vi "GetGlobalDefaultConfiguration.vi"(2 "DO NOT override instruments":bool, 3 "Read defaults?":bool) -> (1 "Configuration File IV":path)   [LabVIEW 2018]
uses:
  QC_MeasurementSetup.vi
  InstrControl/InstrControl.lvclass
panel:
  out "Configuration File Striptest":path
  out "Configuration File Cis":path
  out "Configuration File Stability":path
  out "Configuration File CV":path
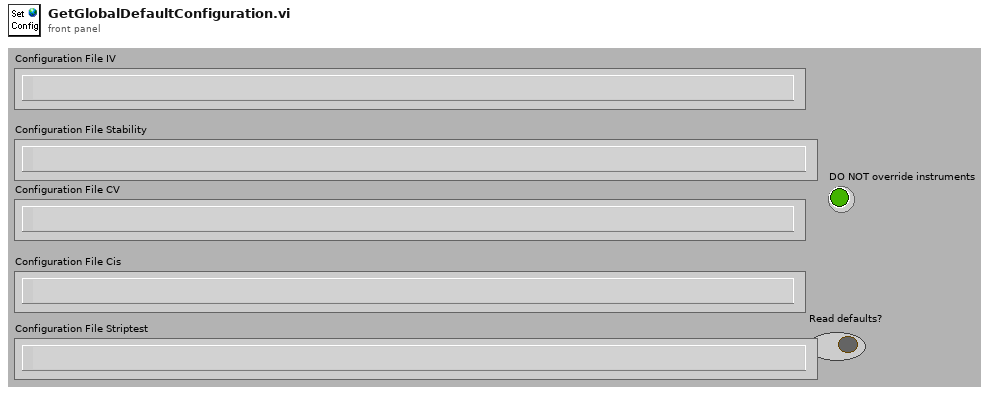
[diagram p1: front panel]
types:
  T1 = cluster{"Supply":refnum<class "SupplyControl.lvclass">, "Initial Voltage [V]":dbl, "Final Voltage [V]":dbl, "Step Size [V]":dbl, "Step Interval [s]":i32, "Number Of Steps":u32, "Ramp down steps [V]":dbl, "Ramp down Interval [s]":i32, "hold steps":i32, "Set Current Limit?":bool, "Current Limit [µA]":dbl, "Temperature Readout":enum16{"Read Arduino", "Enter manually"}, "Arduino":refnum<class "ArduinoControl.lvclass">, "Supply Name":string, "V_breakdown Limit [V]":dbl, "Switching":refnum<class "Switching.lvclass">, "Matrix used?":bool, "Matrix X Channels":cluster{"Bias Supply / SMU LO":i32, "Bias Supply / SMU HI":i32, "CV Box LO":i32, "CV Box HI":i32, "CV Box LO IN":i32, "CV Box HI IN":i32, "Volt meter LO":i32, "Volt meter HI":i32, "Mux1 C1":i32, "Mux1 C2":i32, "Mux2 C1":i32, "Mux2 C2":i32}, "IV Test?":bool}
  T2 = cluster{"Supply":refnum<class "SupplyControl.lvclass">, "LCR":refnum<class "LCRControl.lvclass">, "Initial Voltage [V]":dbl, "Final Voltage [V]":dbl, "Step Size [V]":dbl, "Step Interval [s]":i32, "Number Of Steps":u32, "AC frequency [Hz]":i32, "RC Configuration":u16, "AC amplitude [V]":dbl, "Ramp down steps [V]":dbl, "Ramp down Interval [s]":i32, "Set Current Limit?":bool, "Current Limit [µA]":dbl, "Temperature Readout":enum16{"Read Arduino", "Enter manually"}, "Arduino":refnum<class "ArduinoControl.lvclass">, "Supply Name":string, "LCR Name":string, "V_depletion Limit [V]":dbl, "Switching":refnum<class "Switching.lvclass">, "Matrix used?":bool, "Matrix X Channels":cluster{"Bias Supply / SMU LO":i32, "Bias Supply / SMU HI":i32, "CV Box LO":i32, "CV Box HI":i32, "CV Box LO IN":i32, "CV Box HI IN":i32, "Volt meter LO":i32, "Volt meter HI":i32, "Mux1 C1":i32, "Mux1 C2":i32, "Mux2 C1":i32, "Mux2 C2":i32}, "CV Test?":bool}
  T3 = cluster{"Supply":refnum<class "SupplyControl.lvclass">, "Voltage [V]":dbl, "Measurement Interval [s]":i32, "Test Duration":u32, "Ramp up steps [V]":dbl, "Ramp up Interval [s]":u32, "Ramp down steps [V]":dbl, "Ramp down Interval [s]":i32, "Set Current Limit?":bool, "Current Limit [µA]":dbl, "Temperature Readout":enum16{"Read Arduino", "Enter manually"}, "Arduino":refnum<class "ArduinoControl.lvclass">, "Supply Name":string, "Maximum current fluctuation [%]":dbl, "Switching.lvclass":refnum<class "Switching.lvclass">, "Matrix used?":bool, "Matrix X Channels":cluster{"Bias Supply / SMU LO":i32, "Bias Supply / SMU HI":i32, "CV Box LO":i32, "CV Box HI":i32, "CV Box LO IN":i32, "CV Box HI IN":i32, "Volt meter LO":i32, "Volt meter HI":i32, "Mux1 C1":i32, "Mux1 C2":i32, "Mux2 C1":i32, "Mux2 C2":i32}, "LCS Test?":bool, "Number of Steps":i32}
  T4 = cluster{"Supply":refnum<class "SupplyControl.lvclass">, "LCR":refnum<class "LCRControl.lvclass">, "Initial Voltage [V]":dbl, "Final Voltage [V]":dbl, "Step Size [V]":dbl, "Step Interval [s]":i32, "Number Of Steps":u32, "AC frequency [Hz]":i32, "RC Configuration":u16, "AC amplitude [V]":dbl, "Ramp down steps [V]":dbl, "Ramp down Interval [s]":i32, "Set Current Limit?":bool, "Current Limit [µA]":dbl, "Temperature Readout":enum16{"Read Arduino", "Enter manually"}, "Arduino":refnum<class "ArduinoControl.lvclass">, "Supply Name":string, "LCR Name":string, "C_is Limit [pF/cm]":dbl, "Switching":refnum<class "Switching.lvclass">, "Matrix used?":bool, "Matrix X Channels":cluster{"Bias Supply / SMU LO":i32, "Bias Supply / SMU HI":i32, "CV Box LO":i32, "CV Box HI":i32, "CV Box LO IN":i32, "CV Box HI IN":i32, "Volt meter LO":i32, "Volt meter HI":i32, "Mux1 C1":i32, "Mux1 C2":i32, "Mux2 C1":i32, "Mux2 C2":i32}}
  T5 = cluster{"Bias Supply":refnum<class "SupplyControl.lvclass">, "SMU":refnum<class "SupplyControl.lvclass">, "LCR":refnum<class "LCRControl.lvclass">, "Probe Card Channels":i32, "Bias Voltage [V]":dbl, "First strip":i32, "Last strip":i32, "Base Voltage [V]":dbl, "Base Ramp Step [V]":dbl, "Base Ramp Interval [ms]":u32, "High Voltage [V]":dbl, "High Ramp Step [V]":dbl, "High Ramp Interval [ms]":u32, "AC frequency [Hz]":i32, "AC amplitude [V]":dbl, "RC Configuration":u16, "Single Needle":bool, "Temperature Readout":enum16{"Read Arduino", "Enter manually"}, "Arduino":refnum<class "ArduinoControl.lvclass">, "Fraction of good strips [%]":dbl, "ProbeStation":refnum<class "ProbeStationControl.lvclass">, "Switching":refnum<class "Switching.lvclass">, "Matrix used?":bool, "Matrix X Channels":cluster{"Bias Supply / SMU LO":i32, "Bias Supply / SMU HI":i32, "CV Box LO":i32, "CV Box HI":i32, "CV Box LO IN":i32, "CV Box HI IN":i32, "Volt meter LO":i32, "Volt meter HI":i32, "Mux1 C1":i32, "Mux1 C2":i32, "Mux2 C1":i32, "Mux2 C2":i32}, "Pinholes Y/N":bool, "Capacitance Y/N":bool, "Resistance Y/N":bool, "Bias Supply Name":string, "SMU Name":string, "LCR Name":string}
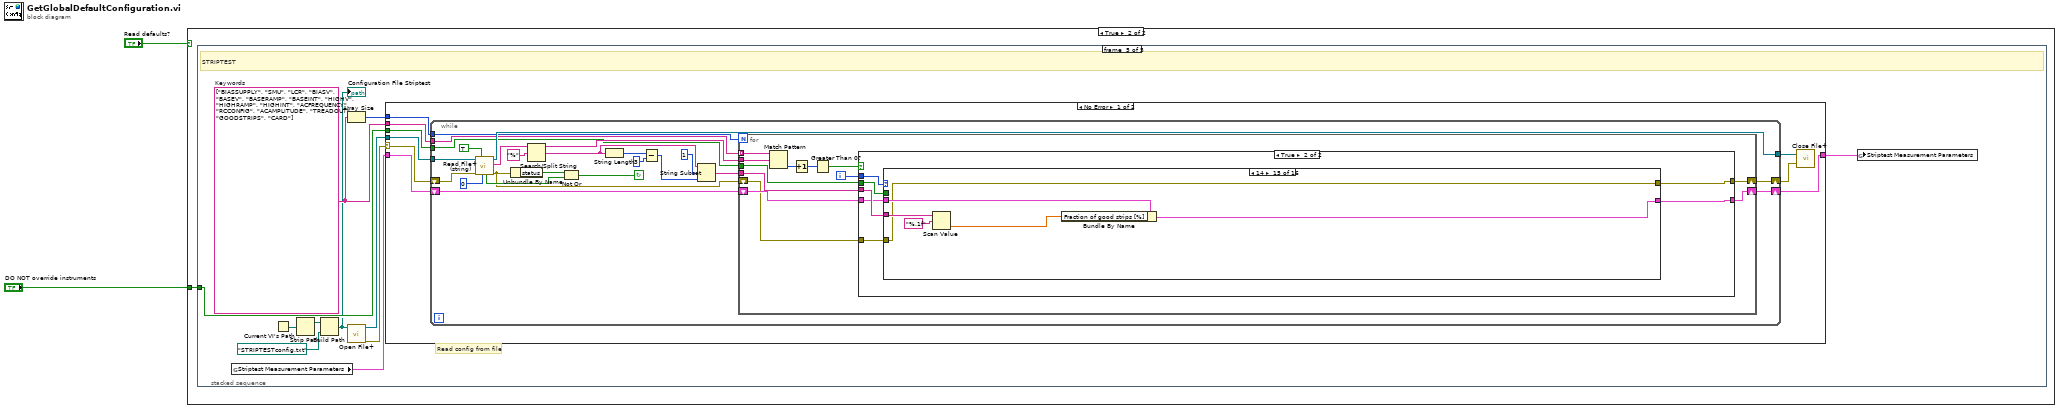
[diagram p0: block diagram]
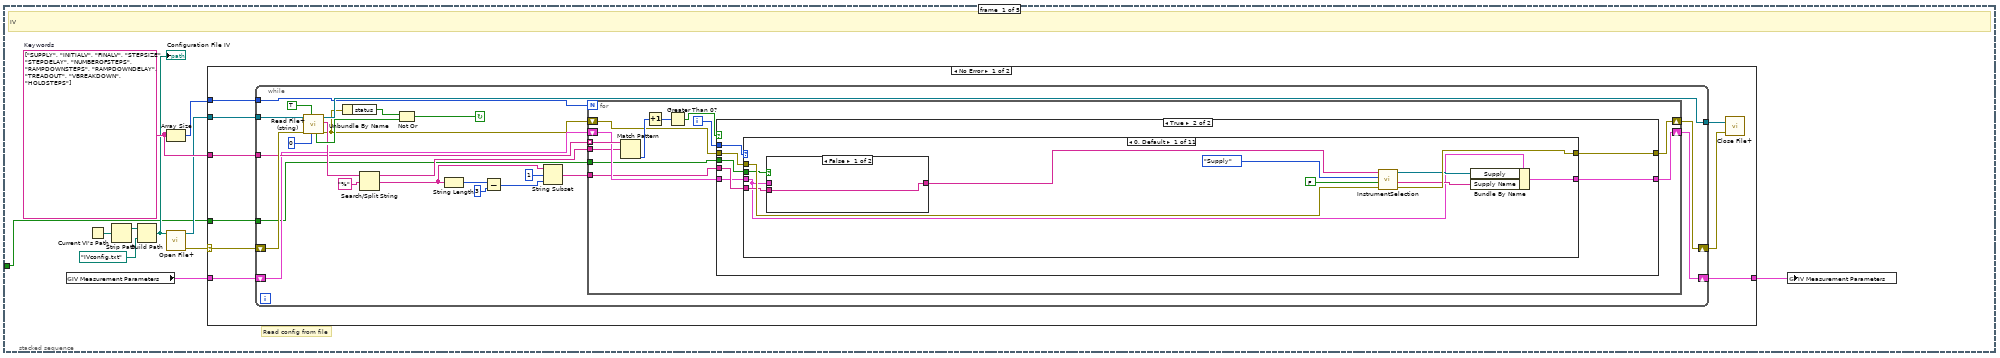
[diagram p3: hidden frame]
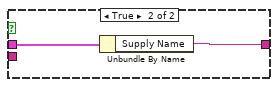
[diagram p5: hidden frame]
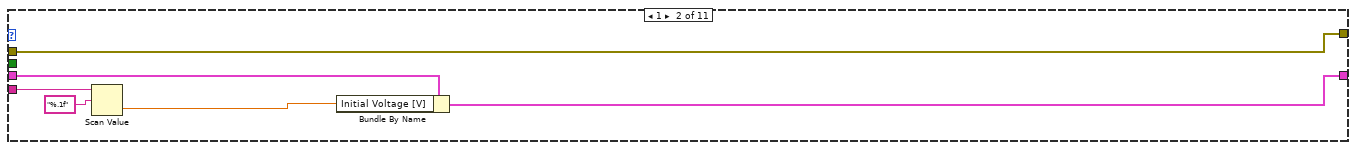
[diagram p6: hidden frame]
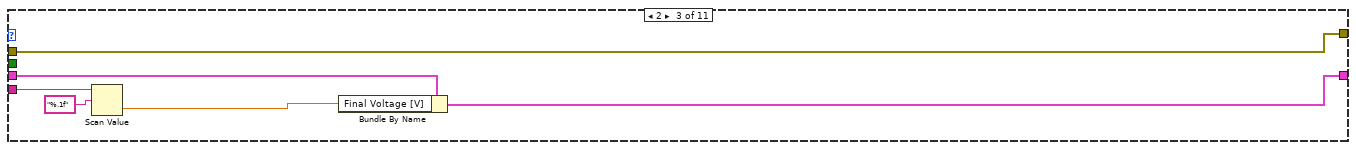
[diagram p7: hidden frame]
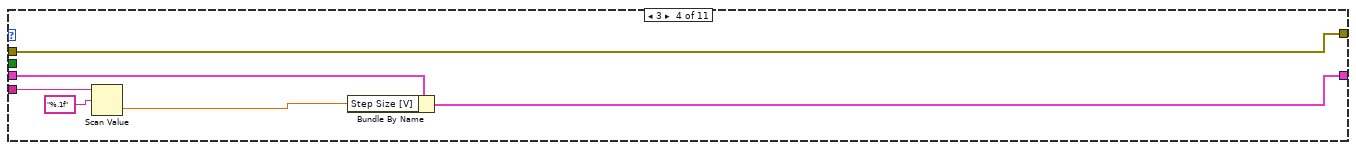
[diagram p8: hidden frame]
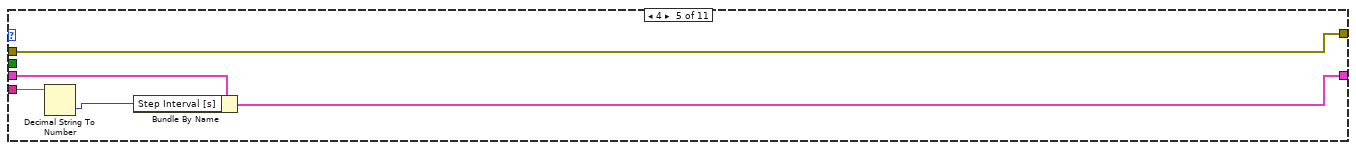
[diagram p9: hidden frame]
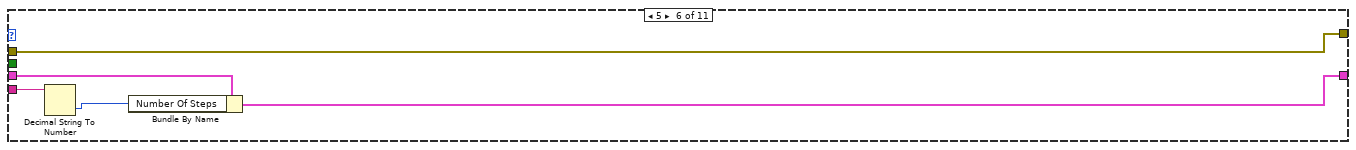
[diagram p10: hidden frame]
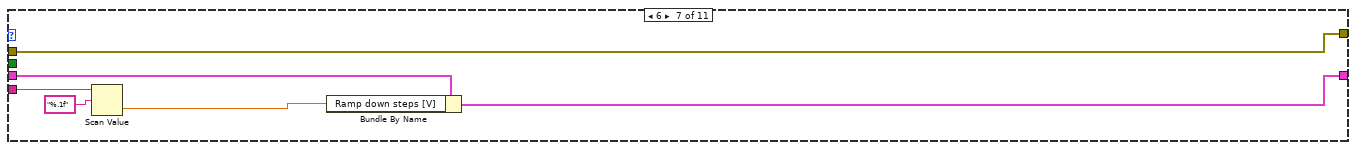
[diagram p11: hidden frame]
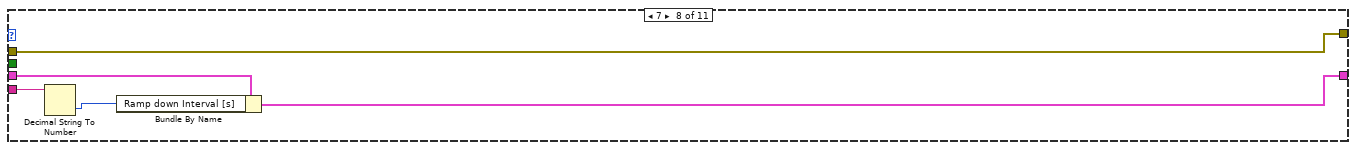
[diagram p12: hidden frame]
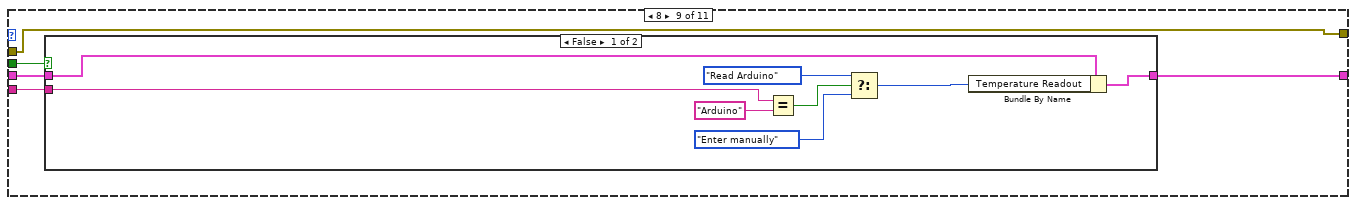
[diagram p13: hidden frame]
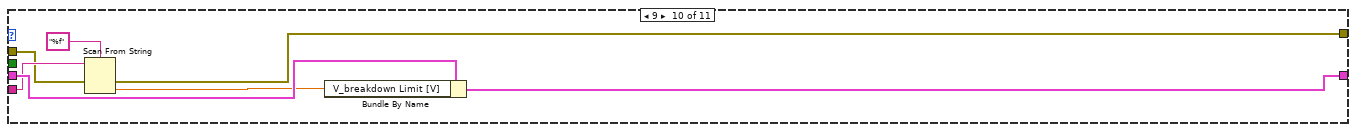
[diagram p15: hidden frame]
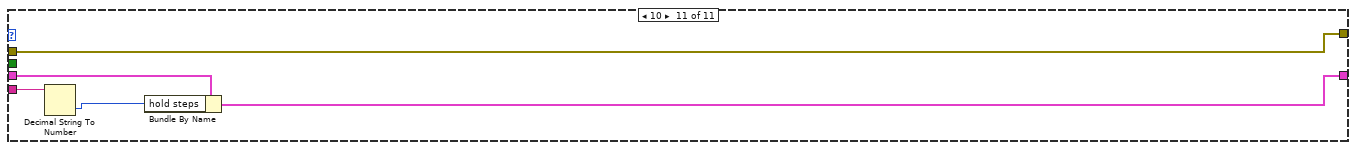
[diagram p16: hidden frame]
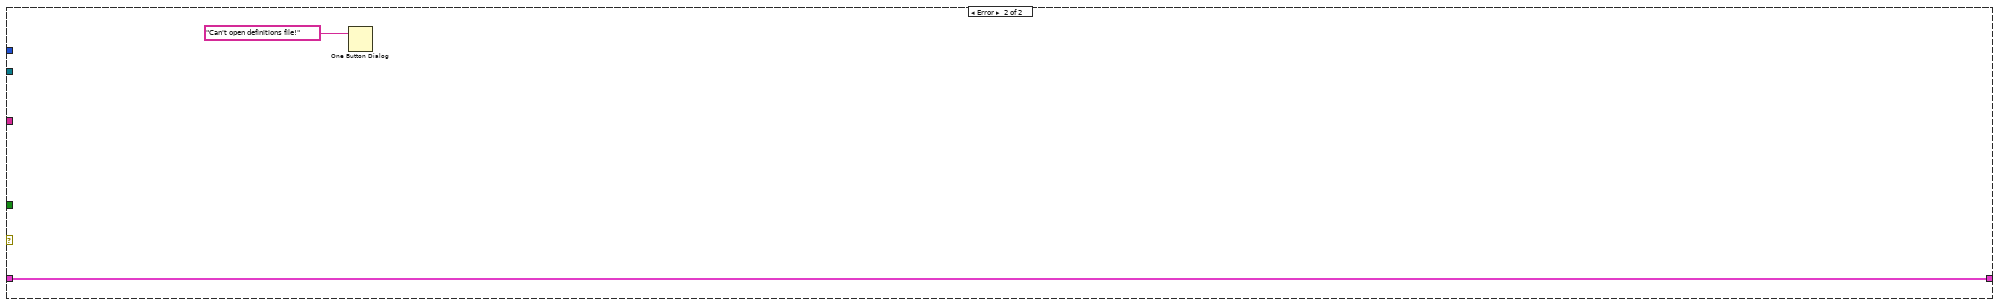
[diagram p17: hidden frame]
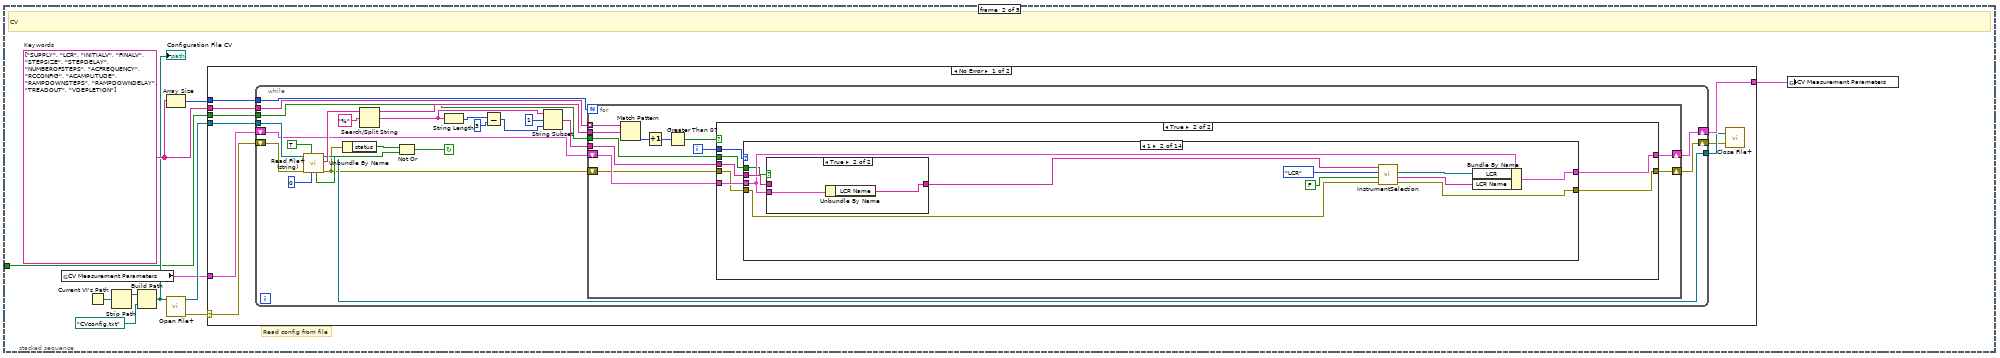
[diagram p18: hidden frame]
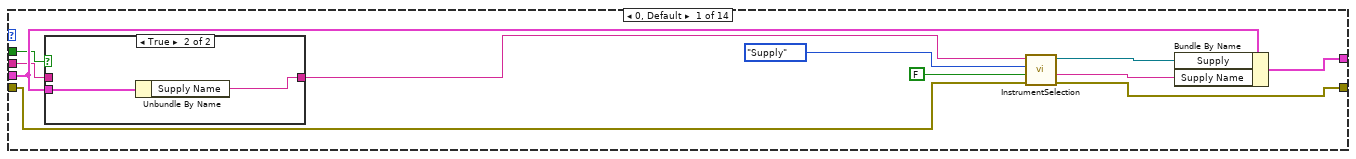
[diagram p20: hidden frame]
diagram:
  n1 = case shown="True" "Read defaults?" {
    tunnel: "DO NOT override instruments" -> [_ w3]
    frame False {
    }
    frame True {
      n2 = stacked-sequence {
        tunnel: w3 -> [w4 w150 w325 w465 w641]
        frame #0 {
          w14 = string[] ["SUPPLY", "INITIALV", "FINALV", "STEPSIZE", "STEPDELAY", "NUMBEROFSTEPS", "RAMPDOWNSTEPS", "RAMPDOWNDELAY", "TREADOUT", "VBREAKDOWN", "HOLDSTEPS"]  # Keywords
          # "Read config from file"
          # "IV"
          n3 = global read "QC_MeasurementSetup.vi" "IV Measurement Parameters"() -> (w5:T1)
          n4 = Current VI's Path() -> (path=w9:path)
          n5 = Strip Path(path=w9) -> (stripped path=w8:path)  [unwired: 1 out]
          n6 = Build Path(base path=w8, name or relative path=path "IVconfig.txt") -> (appended path=w7:path)
          "Configuration File IV" <- w7
          n7 = Array Size(array=w14) -> (size(s)=w13:i32)
          n8 = call <vilib>:"Open File+.vi"("file path (\" \")"=w7) -> ("error out"=w10:errorcluster, "refnum"=w11:refnum<file>)  [unwired: 7 in, 2 out]
          n9 = case shown="No Error" w10 {
            selector: w10 -> [w16 _]
            tunnel: w11 -> [w23 _]
            tunnel: w14 -> [w22 _]
            tunnel: w13 -> [w21 _]
            tunnel: w5 -> [w20 w148]
            tunnel: [w19 w148] -> w6
            tunnel: w4 -> [w15 _]
            frame No Error {
              n10 = while {
                shift-left: w20 -> [w30]
                shift-right: [w28] -> w19
                tunnel: w21 -> [w27]
                tunnel: w22 -> [w33]
                tunnel: [w38] -> w18
                tunnel: w23 -> [w44]
                shift-right: [w25] -> w17
                shift-left: w16 -> [w37]
                tunnel: w15 -> [w24]
                stop <- w40 continue-if-true
                n11 = call <vilib>:"Read File+ (string).vi"("count"=0, "line mode (characters:F)"=TRUE, "error in (no error)"=w37, "refnum"=w44) -> ("error out"=w26:errorcluster, "string"=w39:string, "dup refnum"=w38:refnum<file>, "EOF?"=w42:bool)  [unwired: 3 in, 1 out]
                n12 = Unbundle By Name(w26) -> ("status"=w41:bool)
                n13 = Search/Split String(string=w39, search string/char (-)="%" ("search char (-)")) -> (substring before match=w32:string, match + rest of string=w45:string)  [unwired: 1 in, 1 out]
                n14 = Not Or(1:w42, 2:w41) -> (0:w40:bool)
                n15 = String Length(string=w45) -> (length=w31:i32)
                n16 = Subtract(x=w31, y=3) -> (x-y=w34:i32)
                n17 = String Subset(string=w45, offset (0)=1, length (rest)=w34) -> (substring=w29:string)
                n18 = for {
                  N: w27 -> [_]
                  tunnel: w33 -> [w57] mode=indexing
                  tunnel: w32 -> [w52]
                  shift-right: [w53] -> w28
                  shift-left: w30 -> [w54]
                  tunnel: w29 -> [w51]
                  shift-right: [w49] -> w25
                  shift-left: w26 -> [w50]
                  tunnel: w24 -> [w48]
                  i -> [w55]
                  n19 = Match Pattern(string=w57, regular expression=w52) -> (offset past match=w58:i32)  [unwired: 1 in, 3 out]
                  n20 = Increment(x=w58) -> (x+1=w59:i32)
                  n21 = Greater Than 0?(x=w59) -> (x > 0?=w56:bool)
                  n22 = case shown="True" w56 {
                    tunnel: w55 -> [_ w68]
                    tunnel: w51 -> [_ w67]
                    tunnel: w54 -> [w61 w66]
                    tunnel: [w61 w65] -> w53
                    tunnel: w50 -> [w60 w64]
                    tunnel: [w60 w63] -> w49
                    tunnel: w48 -> [_ w62]
                    frame False {
                    }
                    frame True {
                      n23 = case shown="0, Default" w68 {
                        tunnel: w67 -> [w73 w86 w91 w97 w103 w108 w113 w119 w124 w140 w144]
                        tunnel: w66 -> [w72 w88 w94 w100 w105 w110 w116 w121 w126 w142 w147]
                        tunnel: [w79 w87 w93 w99 w104 w109 w115 w120 w125 w141 w146] -> w65
                        tunnel: w64 -> [w78 w83 w89 w95 w101 w106 w111 w117 w123 w137 w143]
                        tunnel: [w77 w83 w89 w95 w101 w106 w111 w117 w123 w136 w143] -> w63
                        tunnel: w62 -> [w70 _ _ _ _ _ _ _ w122 _ _]
                        frame 0, Default {
                          n24 = case shown="False" w70 {
                            tunnel: w73 -> [w80 _]
                            tunnel: [w80 w81] -> w71
                            tunnel: w72 -> [_ w82]
                            frame False {
                            }
                            frame True {
                              n25 = Unbundle By Name(w82) -> ("Supply Name"=w81:string)
                            }
                          }
                          n26 = call "InstrumentSelection.vi"("error in (no error)"=w78, "Verify GPIB address"=FALSE, "Instrument type"=enum16{"Supply", "LCR", "Multimeter"}."Supply", "Instrument name IN"=w71) -> ("error out"=w77:errorcluster, "Instrument name OUT"=w76:string, "Supply"=w75:refnum<class "SupplyControl.lvclass">)  [unwired: 2 in, 3 out]
                          n27 = Bundle By Name(cluster=w72, "Supply"=w75, "Supply Name"=w76) -> (w79:T1)
                        }
                        frame 1 {
                          n28 = Scan Value(string=w86, format string="%.1f") -> (value=w85:dbl)  [unwired: 1 in, 1 out]
                          n29 = Bundle By Name(cluster=w88, "Initial Voltage [V]"=w85) -> (w87:T1)
                        }
                        frame 2 {
                          n30 = Scan Value(string=w91, format string="%.1f") -> (value=w90:dbl)  [unwired: 1 in, 1 out]
                          n31 = Bundle By Name(cluster=w94, "Final Voltage [V]"=w90) -> (w93:T1)
                        }
                        frame 3 {
                          n32 = Scan Value(string=w97, format string="%.1f") -> (value=w96:dbl)  [unwired: 1 in, 1 out]
                          n33 = Bundle By Name(cluster=w100, "Step Size [V]"=w96) -> (w99:T1)
                        }
                        frame 4 {
                          n34 = Decimal String To Number(string=w103) -> (number=w102:i32)  [unwired: 2 in, 1 out]
                          n35 = Bundle By Name(cluster=w105, "Step Interval [s]"=w102) -> (w104:T1)
                        }
                        frame 5 {
                          n36 = Decimal String To Number(string=w108) -> (number=w107:i32)  [unwired: 2 in, 1 out]
                          n37 = Bundle By Name(cluster=w110, "Number Of Steps"=w107) -> (w109:T1)
                        }
                        frame 6 {
                          n38 = Scan Value(string=w113, format string="%.1f") -> (value=w112:dbl)  [unwired: 1 in, 1 out]
                          n39 = Bundle By Name(cluster=w116, "Ramp down steps [V]"=w112) -> (w115:T1)
                        }
                        frame 7 {
                          n40 = Decimal String To Number(string=w119) -> (number=w118:i32)  [unwired: 2 in, 1 out]
                          n41 = Bundle By Name(cluster=w121, "Ramp down Interval [s]"=w118) -> (w120:T1)
                        }
                        frame 8 {
                          n42 = case shown="False" w122 {
                            tunnel: w126 -> [w134 w135]
                            tunnel: [w133 w135] -> w125
                            tunnel: w124 -> [w132 _]
                            frame False {
                              n43 = Equal?(x=w132, y="Arduino") -> (x = y?=w130:bool)
                              n44 = Select(t=enum16{"Read Arduino", "Enter manually"}."Read Arduino" ("Temperature Readout"), s=w130, f=enum16{"Read Arduino", "Enter manually"}."Enter manually" ("Temperature Readout")) -> (s? t:f=w127:enum16{"Read Arduino", "Enter manually"})
                              n45 = Bundle By Name(cluster=w134, "Temperature Readout"=w127) -> (w133:T1)
                            }
                            frame True {
                            }
                          }
                        }
                        frame 9 {
                          n46 = Scan From String(format string="%f", input string=w140, error in=w137) -> (error out=w136:errorcluster, output 1=w139:dbl)  [unwired: 2 in, 2 out]
                          n47 = Bundle By Name(cluster=w142, "V_breakdown Limit [V]"=w139) -> (w141:T1)
                        }
                        frame 10 {
                          n48 = Decimal String To Number(string=w144) -> (number=w145:i32)  [unwired: 2 in, 1 out]
                          n49 = Bundle By Name(cluster=w147, "hold steps"=w145) -> (w146:T1)
                        }
                      }
                    }
                  }
                }
              }
              n50 = call <vilib>:"Close File+.vi"("error in (no error)"=w17, "refnum"=w18) -> ()  [unwired: 3 in, 3 out]
            }
            frame Error {
              n51 = One Button Dialog(message="Can't open definitions file!") -> ()  [unwired: 1 in, 1 out]
            }
          }
          n52 = global write "QC_MeasurementSetup.vi" "IV Measurement Parameters"(w6) -> ()
        }
        frame #1 {
          w160 = string[] ["SUPPLY", "LCR", "INITIALV", "FINALV", "STEPSIZE", "STEPDELAY", "NUMBEROFSTEPS", "ACFREQUENCY", "RCCONFIG", "ACAMPLITUDE", "RAMPDOWNSTEPS", "RAMPDOWNDELAY", "TREADOUT", "VDEPLETION"]  # Keywords
          # "Read config from file"
          # "CV"
          n53 = global read "QC_MeasurementSetup.vi" "CV Measurement Parameters"() -> (w151:T2)
          n54 = Current VI's Path() -> (path=w155:path)
          n55 = Strip Path(path=w155) -> (stripped path=w154:path)  [unwired: 1 out]
          n56 = Build Path(base path=w154, name or relative path=path "CVconfig.txt") -> (appended path=w153:path)
          "Configuration File CV" <- w153
          n57 = Array Size(array=w160) -> (size(s)=w159:i32)
          n58 = call <vilib>:"Open File+.vi"("file path (\" \")"=w153) -> ("error out"=w156:errorcluster, "refnum"=w157:refnum<file>)  [unwired: 7 in, 2 out]
          n59 = case shown="No Error" w156 {
            selector: w156 -> [w162 _]
            tunnel: w157 -> [w169 _]
            tunnel: w160 -> [w168 _]
            tunnel: w159 -> [w167 _]
            tunnel: w151 -> [w166 w323]
            tunnel: [w165 w323] -> w152
            tunnel: w150 -> [w161 _]
            frame No Error {
              n60 = while {
                shift-left: w166 -> [w176]
                shift-right: [w174] -> w165
                tunnel: w167 -> [w173]
                tunnel: w168 -> [w179]
                tunnel: [w184] -> w164
                tunnel: w169 -> [w190]
                shift-right: [w171] -> w163
                shift-left: w162 -> [w183]
                tunnel: w161 -> [w170]
                stop <- w186 continue-if-true
                n61 = call <vilib>:"Read File+ (string).vi"("count"=0, "line mode (characters:F)"=TRUE, "error in (no error)"=w183, "refnum"=w190) -> ("error out"=w172:errorcluster, "string"=w185:string, "dup refnum"=w184:refnum<file>, "EOF?"=w188:bool)  [unwired: 3 in, 1 out]
                n62 = Unbundle By Name(w172) -> ("status"=w187:bool)
                n63 = Search/Split String(string=w185, search string/char (-)="%" ("search char (-)")) -> (substring before match=w178:string, match + rest of string=w191:string)  [unwired: 1 in, 1 out]
                n64 = Not Or(1:w188, 2:w187) -> (0:w186:bool)
                n65 = String Length(string=w191) -> (length=w177:i32)
                n66 = Subtract(x=w177, y=3) -> (x-y=w180:i32)
                n67 = String Subset(string=w191, offset (0)=1, length (rest)=w180) -> (substring=w175:string)
                n68 = for {
                  N: w173 -> [_]
                  tunnel: w179 -> [w203] mode=indexing
                  tunnel: w178 -> [w198]
                  shift-right: [w199] -> w174
                  shift-left: w176 -> [w200]
                  tunnel: w175 -> [w197]
                  shift-right: [w195] -> w171
                  shift-left: w172 -> [w196]
                  tunnel: w170 -> [w194]
                  i -> [w201]
                  n69 = Match Pattern(string=w203, regular expression=w198) -> (offset past match=w204:i32)  [unwired: 1 in, 3 out]
                  n70 = Increment(x=w204) -> (x+1=w205:i32)
                  n71 = Greater Than 0?(x=w205) -> (x > 0?=w202:bool)
                  n72 = case shown="True" w202 {
                    tunnel: w201 -> [_ w214]
                    tunnel: w197 -> [_ w213]
                    tunnel: w200 -> [w207 w212]
                    tunnel: [w207 w211] -> w199
                    tunnel: w196 -> [w206 w210]
                    tunnel: [w206 w209] -> w195
                    tunnel: w194 -> [_ w208]
                    frame False {
                    }
                    frame True {
                      n73 = case shown="1" w214 {
                        tunnel: w213 -> [w218 w233 w246 w251 w257 w263 w268 w273 w281 w290 w293 w299 w304 w320]
                        tunnel: w212 -> [w219 w232 w248 w254 w260 w265 w270 w275 w284 w288 w296 w301 w306 w316]
                        tunnel: [w225 w239 w247 w253 w259 w264 w269 w274 w283 w286 w295 w300 w305 w317] -> w211
                        tunnel: w210 -> [w223 w238 w243 w249 w255 w261 w266 w271 w276 w285 w291 w297 w303 w319]
                        tunnel: [w224 w237 w243 w249 w255 w261 w266 w271 w276 w285 w291 w297 w303 w318] -> w209
                        tunnel: w208 -> [w216 w230 _ _ _ _ _ _ _ _ _ _ w302 _]
                        frame 0, Default {
                          n74 = case shown="True" w216 {
                            tunnel: w218 -> [w226 _]
                            tunnel: [w226 w227] -> w217
                            tunnel: w219 -> [_ w228]
                            frame False {
                            }
                            frame True {
                              n75 = Unbundle By Name(w228) -> ("Supply Name"=w227:string)
                            }
                          }
                          n76 = call "InstrumentSelection.vi"("error in (no error)"=w223, "Verify GPIB address"=FALSE, "Instrument type"=enum16{"Supply", "LCR", "Multimeter"}."Supply", "Instrument name IN"=w217) -> ("error out"=w224:errorcluster, "Instrument name OUT"=w221:string, "Supply"=w222:refnum<class "SupplyControl.lvclass">)  [unwired: 2 in, 3 out]
                          n77 = Bundle By Name(cluster=w219, "Supply"=w222, "Supply Name"=w221) -> (w225:T2)
                        }
                        frame 1 {
                          n78 = case shown="True" w230 {
                            tunnel: w233 -> [w240 _]
                            tunnel: [w240 w241] -> w231
                            tunnel: w232 -> [_ w242]
                            frame False {
                            }
                            frame True {
                              n79 = Unbundle By Name(w242) -> ("LCR Name"=w241:string)
                            }
                          }
                          n80 = call "InstrumentSelection.vi"("error in (no error)"=w238, "Verify GPIB address"=FALSE, "Instrument type"=enum16{"Supply", "LCR", "Multimeter"}."LCR", "Instrument name IN"=w231) -> ("error out"=w237:errorcluster, "Instrument name OUT"=w236:string, "LCR"=w235:refnum<class "LCRControl.lvclass">)  [unwired: 2 in, 3 out]
                          n81 = Bundle By Name(cluster=w232, "LCR"=w235, "LCR Name"=w236) -> (w239:T2)
                        }
                        frame 2 {
                          n82 = Scan Value(string=w246, format string="%.1f") -> (value=w245:dbl)  [unwired: 1 in, 1 out]
                          n83 = Bundle By Name(cluster=w248, "Initial Voltage [V]"=w245) -> (w247:T2)
                        }
                        frame 3 {
                          n84 = Scan Value(string=w251, format string="%.1f") -> (value=w250:dbl)  [unwired: 1 in, 1 out]
                          n85 = Bundle By Name(cluster=w254, "Final Voltage [V]"=w250) -> (w253:T2)
                        }
                        frame 4 {
                          n86 = Scan Value(string=w257, format string="%.1f") -> (value=w256:dbl)  [unwired: 1 in, 1 out]
                          n87 = Bundle By Name(cluster=w260, "Step Size [V]"=w256) -> (w259:T2)
                        }
                        frame 5 {
                          n88 = Decimal String To Number(string=w263) -> (number=w262:i32)  [unwired: 2 in, 1 out]
                          n89 = Bundle By Name(cluster=w265, "Step Interval [s]"=w262) -> (w264:T2)
                        }
                        frame 6 {
                          n90 = Decimal String To Number(string=w268) -> (number=w267:i32)  [unwired: 2 in, 1 out]
                          n91 = Bundle By Name(cluster=w270, "Number Of Steps"=w267) -> (w269:T2)
                        }
                        frame 7 {
                          n92 = Decimal String To Number(string=w273) -> (number=w272:i32)  [unwired: 2 in, 1 out]
                          n93 = Bundle By Name(cluster=w275, "AC frequency [Hz]"=w272) -> (w274:T2)
                        }
                        frame 8 {
                          w280 = u16 0 items=["serial", "parallel"] ("RC Configuration")
                          w279 = u16 1 items=["serial", "parallel"] ("RC Configuration")
                          n94 = Equal?(x=w281, y="serial") -> (x = y?=w278:bool)
                          n95 = Select(t=w280, s=w278, f=w279) -> (s? t:f=w277:u16)
                          n96 = Bundle By Name(cluster=w284, "RC Configuration"=w277) -> (w283:T2)
                        }
                        frame 9 {
                          n97 = Scan Value(string=w290, format string="%.1f") -> (value=w287:dbl)  [unwired: 1 in, 1 out]
                          n98 = Bundle By Name(cluster=w288, "AC amplitude [V]"=w287) -> (w286:T2)
                        }
                        frame 10 {
                          n99 = Scan Value(string=w293, format string="%.1f") -> (value=w292:dbl)  [unwired: 1 in, 1 out]
                          n100 = Bundle By Name(cluster=w296, "Ramp down steps [V]"=w292) -> (w295:T2)
                        }
                        frame 11 {
                          n101 = Decimal String To Number(string=w299) -> (number=w298:i32)  [unwired: 2 in, 1 out]
                          n102 = Bundle By Name(cluster=w301, "Ramp down Interval [s]"=w298) -> (w300:T2)
                        }
                        frame 12 {
                          n103 = case shown="False" w302 {
                            tunnel: w306 -> [w314 w315]
                            tunnel: [w313 w315] -> w305
                            tunnel: w304 -> [w312 _]
                            frame False {
                              n104 = Equal?(x=w312, y="Arduino") -> (x = y?=w310:bool)
                              n105 = Select(t=enum16{"Read Arduino", "Enter manually"}."Read Arduino" ("Temperature Readout"), s=w310, f=enum16{"Read Arduino", "Enter manually"}."Enter manually" ("Temperature Readout")) -> (s? t:f=w307:enum16{"Read Arduino", "Enter manually"})
                              n106 = Bundle By Name(cluster=w314, "Temperature Readout"=w307) -> (w313:T2)
                            }
                            frame True {
                            }
                          }
                        }
                        frame 13 {
                          n107 = Scan From String(format string="%f", input string=w320, error in=w319) -> (error out=w318:errorcluster, output 1=w322:dbl)  [unwired: 2 in, 2 out]
                          n108 = Bundle By Name(cluster=w316, "V_depletion Limit [V]"=w322) -> (w317:T2)
                        }
                      }
                    }
                  }
                }
              }
              n109 = call <vilib>:"Close File+.vi"("error in (no error)"=w163, "refnum"=w164) -> ()  [unwired: 3 in, 3 out]
            }
            frame Error {
              n110 = One Button Dialog(message="Can't open definitions file!") -> ()  [unwired: 1 in, 1 out]
            }
          }
          n111 = global write "QC_MeasurementSetup.vi" "CV Measurement Parameters"(w152) -> ()
        }
        frame #2 {
          w335 = string[] ["SUPPLY", "VOLTAGE", "INTERVAL", "DURATION", "RAMPUPSTEPS", "RAMPUPDELAY", "RAMPDOWNSTEPS", "RAMPDOWNDELAY", "TREADOUT", "IFLUCTUATIONS"]  # Keywords
          # "Read config from file"
          # "STABILITY"
          n112 = global read "QC_MeasurementSetup.vi" "Current Stability Measurement Parameters"() -> (w326:T3)
          n113 = Current VI's Path() -> (path=w330:path)
          n114 = Strip Path(path=w330) -> (stripped path=w329:path)  [unwired: 1 out]
          n115 = Build Path(base path=w329, name or relative path=path "STABILITYconfig.txt") -> (appended path=w328:path)
          "Configuration File Stability" <- w328
          n116 = Array Size(array=w335) -> (size(s)=w334:i32)
          n117 = call <vilib>:"Open File+.vi"("file path (\" \")"=w328) -> ("error out"=w331:errorcluster, "refnum"=w332:refnum<file>)  [unwired: 7 in, 2 out]
          n118 = case shown="No Error" w331 {
            selector: w331 -> [w337 _]
            tunnel: w332 -> [w344 _]
            tunnel: w335 -> [w343 _]
            tunnel: w334 -> [w342 _]
            tunnel: w326 -> [w341 w463]
            tunnel: [w340 w463] -> w327
            tunnel: w325 -> [w336 _]
            frame No Error {
              n119 = while {
                shift-left: w341 -> [w351]
                shift-right: [w349] -> w340
                tunnel: w342 -> [w348]
                tunnel: w343 -> [w354]
                tunnel: [w359] -> w339
                tunnel: w344 -> [w365]
                shift-right: [w346] -> w338
                shift-left: w337 -> [w358]
                tunnel: w336 -> [w345]
                stop <- w361 continue-if-true
                n120 = call <vilib>:"Read File+ (string).vi"("count"=0, "line mode (characters:F)"=TRUE, "error in (no error)"=w358, "refnum"=w365) -> ("error out"=w347:errorcluster, "string"=w360:string, "dup refnum"=w359:refnum<file>, "EOF?"=w363:bool)  [unwired: 3 in, 1 out]
                n121 = Unbundle By Name(w347) -> ("status"=w362:bool)
                n122 = Search/Split String(string=w360, search string/char (-)="%" ("search char (-)")) -> (substring before match=w353:string, match + rest of string=w366:string)  [unwired: 1 in, 1 out]
                n123 = Not Or(1:w363, 2:w362) -> (0:w361:bool)
                n124 = String Length(string=w366) -> (length=w352:i32)
                n125 = Subtract(x=w352, y=3) -> (x-y=w355:i32)
                n126 = String Subset(string=w366, offset (0)=1, length (rest)=w355) -> (substring=w350:string)
                n127 = for {
                  N: w348 -> [_]
                  tunnel: w354 -> [w378] mode=indexing
                  tunnel: w353 -> [w373]
                  shift-right: [w374] -> w349
                  shift-left: w351 -> [w375]
                  tunnel: w350 -> [w372]
                  shift-right: [w370] -> w346
                  shift-left: w347 -> [w371]
                  tunnel: w345 -> [w369]
                  i -> [w376]
                  n128 = Match Pattern(string=w378, regular expression=w373) -> (offset past match=w379:i32)  [unwired: 1 in, 3 out]
                  n129 = Increment(x=w379) -> (x+1=w380:i32)
                  n130 = Greater Than 0?(x=w380) -> (x > 0?=w377:bool)
                  n131 = case shown="True" w377 {
                    tunnel: w376 -> [_ w389]
                    tunnel: w372 -> [_ w388]
                    tunnel: w375 -> [w382 w387]
                    tunnel: [w382 w386] -> w374
                    tunnel: w371 -> [w381 w385]
                    tunnel: [w381 w384] -> w370
                    tunnel: w369 -> [_ w383]
                    frame False {
                    }
                    frame True {
                      n132 = case shown="0, Default" w389 {
                        tunnel: w388 -> [w394 w407 w411 w416 w422 w428 w433 w439 w444 w459]
                        tunnel: w387 -> [w391 w409 w414 w419 w425 w430 w436 w441 w446 w460]
                        tunnel: [w400 w408 w413 w418 w424 w429 w435 w440 w445 w458] -> w386
                        tunnel: w385 -> [w399 w404 w412 w417 w423 w426 w431 w437 w443 w456]
                        tunnel: [w398 w404 w412 w417 w423 w426 w431 w437 w443 w457] -> w384
                        tunnel: w383 -> [w392 _ _ _ _ _ _ _ w442 _]
                        frame 0, Default {
                          n133 = case shown="True" w392 {
                            tunnel: w394 -> [w401 _]
                            tunnel: [w401 w402] -> w393
                            tunnel: w391 -> [_ w403]
                            frame False {
                            }
                            frame True {
                              n134 = Unbundle By Name(w403) -> ("Supply Name"=w402:string)
                            }
                          }
                          n135 = call "InstrumentSelection.vi"("error in (no error)"=w399, "Verify GPIB address"=FALSE, "Instrument type"=enum16{"Supply", "LCR", "Multimeter"}."Supply", "Instrument name IN"=w393) -> ("error out"=w398:errorcluster, "Instrument name OUT"=w397:string, "Supply"=w396:refnum<class "SupplyControl.lvclass">)  [unwired: 2 in, 3 out]
                          n136 = Bundle By Name(cluster=w391, "Supply"=w396, "Supply Name"=w397) -> (w400:T3)
                        }
                        frame 1 {
                          n137 = Scan Value(string=w407, format string="%.1f") -> (value=w406:dbl)  [unwired: 1 in, 1 out]
                          n138 = Bundle By Name(cluster=w409, "Voltage [V]"=w406) -> (w408:T3)
                        }
                        frame 2 {
                          n139 = Decimal String To Number(string=w411) -> (number=w410:i32)  [unwired: 2 in, 1 out]
                          n140 = Bundle By Name(cluster=w414, "Measurement Interval [s]"=w410) -> (w413:T3)
                        }
                        frame 3 {
                          n141 = Decimal String To Number(string=w416) -> (number=w415:i32)  [unwired: 2 in, 1 out]
                          n142 = Bundle By Name(cluster=w419, "Test Duration"=w415) -> (w418:T3)
                        }
                        frame 4 {
                          n143 = Scan Value(string=w422, format string="%.1f") -> (value=w420:dbl)  [unwired: 1 in, 1 out]
                          n144 = Bundle By Name(cluster=w425, "Ramp up steps [V]"=w420) -> (w424:T3)
                        }
                        frame 5 {
                          n145 = Decimal String To Number(string=w428) -> (number=w427:i32)  [unwired: 2 in, 1 out]
                          n146 = Bundle By Name(cluster=w430, "Ramp up Interval [s]"=w427) -> (w429:T3)
                        }
                        frame 6 {
                          n147 = Scan Value(string=w433, format string="%.1f") -> (value=w432:dbl)  [unwired: 1 in, 1 out]
                          n148 = Bundle By Name(cluster=w436, "Ramp down steps [V]"=w432) -> (w435:T3)
                        }
                        frame 7 {
                          n149 = Decimal String To Number(string=w439) -> (number=w438:i32)  [unwired: 2 in, 1 out]
                          n150 = Bundle By Name(cluster=w441, "Ramp down Interval [s]"=w438) -> (w440:T3)
                        }
                        frame 8 {
                          n151 = case shown="False" w442 {
                            tunnel: w446 -> [w454 w455]
                            tunnel: [w453 w455] -> w445
                            tunnel: w444 -> [w452 _]
                            frame False {
                              n152 = Equal?(x=w452, y="Arduino") -> (x = y?=w450:bool)
                              n153 = Select(t=enum16{"Read Arduino", "Enter manually"}."Read Arduino" ("Temperature Readout"), s=w450, f=enum16{"Read Arduino", "Enter manually"}."Enter manually" ("Temperature Readout")) -> (s? t:f=w447:enum16{"Read Arduino", "Enter manually"})
                              n154 = Bundle By Name(cluster=w454, "Temperature Readout"=w447) -> (w453:T3)
                            }
                            frame True {
                            }
                          }
                        }
                        frame 9 {
                          n155 = Scan From String(format string="%f", input string=w459, error in=w456) -> (error out=w457:errorcluster, output 1=w462:dbl)  [unwired: 2 in, 2 out]
                          n156 = Bundle By Name(cluster=w460, "Maximum current fluctuation [%]"=w462) -> (w458:T3)
                        }
                      }
                    }
                  }
                }
              }
              n157 = call <vilib>:"Close File+.vi"("error in (no error)"=w338, "refnum"=w339) -> ()  [unwired: 3 in, 3 out]
            }
            frame Error {
              n158 = One Button Dialog(message="Can't open definitions file!") -> ()  [unwired: 1 in, 1 out]
            }
          }
          n159 = global write "QC_MeasurementSetup.vi" "Current Stability Measurement Parameters"(w327) -> ()
        }
        frame #3 {
          w475 = string[] ["SUPPLY", "LCR", "INITIALV", "FINALV", "STEPSIZE", "STEPDELAY", "NUMBEROFSTEPS", "ACFREQUENCY", "RCCONFIG", "ACAMPLITUDE", "RAMPDOWNSTEPS", "RAMPDOWNDELAY", "TREADOUT", "CISLIMIT"]  # Keywords
          # "Read config from file"
          # "CIS"
          n160 = global read "QC_MeasurementSetup.vi" "Cis Measurement Parameters"() -> (w466:T4)
          n161 = Current VI's Path() -> (path=w470:path)
          n162 = Strip Path(path=w470) -> (stripped path=w469:path)  [unwired: 1 out]
          n163 = Build Path(base path=w469, name or relative path=path "CISconfig.txt") -> (appended path=w468:path)
          "Configuration File Cis" <- w468
          n164 = Array Size(array=w475) -> (size(s)=w474:i32)
          n165 = call <vilib>:"Open File+.vi"("file path (\" \")"=w468) -> ("error out"=w471:errorcluster, "refnum"=w472:refnum<file>)  [unwired: 7 in, 2 out]
          n166 = case shown="No Error" w471 {
            selector: w471 -> [w477 _]
            tunnel: w472 -> [w484 _]
            tunnel: w475 -> [w483 _]
            tunnel: w474 -> [w482 _]
            tunnel: w466 -> [w481 w638]
            tunnel: [w480 w638] -> w467
            tunnel: w465 -> [w476 _]
            frame No Error {
              n167 = while {
                shift-left: w481 -> [w491]
                shift-right: [w489] -> w480
                tunnel: w482 -> [w488]
                tunnel: w483 -> [w494]
                tunnel: [w499] -> w479
                tunnel: w484 -> [w505]
                shift-right: [w486] -> w478
                shift-left: w477 -> [w498]
                tunnel: w476 -> [w485]
                stop <- w501 continue-if-true
                n168 = call <vilib>:"Read File+ (string).vi"("count"=0, "line mode (characters:F)"=TRUE, "error in (no error)"=w498, "refnum"=w505) -> ("error out"=w487:errorcluster, "string"=w500:string, "dup refnum"=w499:refnum<file>, "EOF?"=w503:bool)  [unwired: 3 in, 1 out]
                n169 = Unbundle By Name(w487) -> ("status"=w502:bool)
                n170 = Search/Split String(string=w500, search string/char (-)="%" ("search char (-)")) -> (substring before match=w493:string, match + rest of string=w506:string)  [unwired: 1 in, 1 out]
                n171 = Not Or(1:w503, 2:w502) -> (0:w501:bool)
                n172 = String Length(string=w506) -> (length=w492:i32)
                n173 = Subtract(x=w492, y=3) -> (x-y=w495:i32)
                n174 = String Subset(string=w506, offset (0)=1, length (rest)=w495) -> (substring=w490:string)
                n175 = for {
                  N: w488 -> [_]
                  tunnel: w494 -> [w518] mode=indexing
                  tunnel: w493 -> [w513]
                  shift-right: [w514] -> w489
                  shift-left: w491 -> [w515]
                  tunnel: w490 -> [w512]
                  shift-right: [w510] -> w486
                  shift-left: w487 -> [w511]
                  tunnel: w485 -> [w509]
                  i -> [w516]
                  n176 = Match Pattern(string=w518, regular expression=w513) -> (offset past match=w519:i32)  [unwired: 1 in, 3 out]
                  n177 = Increment(x=w519) -> (x+1=w520:i32)
                  n178 = Greater Than 0?(x=w520) -> (x > 0?=w517:bool)
                  n179 = case shown="True" w517 {
                    tunnel: w516 -> [_ w529]
                    tunnel: w512 -> [_ w528]
                    tunnel: w515 -> [w522 w527]
                    tunnel: [w522 w526] -> w514
                    tunnel: w511 -> [w521 w525]
                    tunnel: [w521 w524] -> w510
                    tunnel: w509 -> [_ w523]
                    frame False {
                    }
                    frame True {
                      n180 = case shown="9" w529 {
                        tunnel: w528 -> [w534 w548 w561 w566 w572 w578 w583 w588 w596 w605 w608 w614 w619 w635]
                        tunnel: w527 -> [w532 w547 w563 w569 w575 w580 w585 w590 w599 w603 w611 w616 w621 w634]
                        tunnel: [w540 w554 w562 w568 w574 w579 w584 w589 w598 w601 w610 w615 w620 w633] -> w526
                        tunnel: w525 -> [w538 w553 w558 w564 w570 w576 w581 w586 w591 w600 w606 w612 w618 w631]
                        tunnel: [w539 w552 w558 w564 w570 w576 w581 w586 w591 w600 w606 w612 w618 w632] -> w524
                        tunnel: w523 -> [w531 w545 _ _ _ _ _ _ _ _ _ _ w617 _]
                        frame 0, Default {
                          n181 = case shown="True" w531 {
                            tunnel: w534 -> [w541 _]
                            tunnel: [w541 w542] -> w533
                            tunnel: w532 -> [_ w543]
                            frame False {
                            }
                            frame True {
                              n182 = Unbundle By Name(w543) -> ("Supply Name"=w542:string)
                            }
                          }
                          n183 = call "InstrumentSelection.vi"("error in (no error)"=w538, "Verify GPIB address"=FALSE, "Instrument type"=enum16{"Supply", "LCR", "Multimeter"}."Supply", "Instrument name IN"=w533) -> ("error out"=w539:errorcluster, "Instrument name OUT"=w536:string, "Supply"=w537:refnum<class "SupplyControl.lvclass">)  [unwired: 2 in, 3 out]
                          n184 = Bundle By Name(cluster=w532, "Supply"=w537, "Supply Name"=w536) -> (w540:T4)
                        }
                        frame 1 {
                          n185 = case shown="True" w545 {
                            tunnel: w548 -> [w555 _]
                            tunnel: [w555 w556] -> w546
                            tunnel: w547 -> [_ w557]
                            frame False {
                            }
                            frame True {
                              n186 = Unbundle By Name(w557) -> ("LCR Name"=w556:string)
                            }
                          }
                          n187 = call "InstrumentSelection.vi"("error in (no error)"=w553, "Verify GPIB address"=FALSE, "Instrument type"=enum16{"Supply", "LCR", "Multimeter"}."LCR", "Instrument name IN"=w546) -> ("error out"=w552:errorcluster, "Instrument name OUT"=w551:string, "LCR"=w550:refnum<class "LCRControl.lvclass">)  [unwired: 2 in, 3 out]
                          n188 = Bundle By Name(cluster=w547, "LCR"=w550, "LCR Name"=w551) -> (w554:T4)
                        }
                        frame 2 {
                          n189 = Scan Value(string=w561, format string="%.1f") -> (value=w560:dbl)  [unwired: 1 in, 1 out]
                          n190 = Bundle By Name(cluster=w563, "Initial Voltage [V]"=w560) -> (w562:T4)
                        }
                        frame 3 {
                          n191 = Scan Value(string=w566, format string="%.1f") -> (value=w565:dbl)  [unwired: 1 in, 1 out]
                          n192 = Bundle By Name(cluster=w569, "Final Voltage [V]"=w565) -> (w568:T4)
                        }
                        frame 4 {
                          n193 = Scan Value(string=w572, format string="%.1f") -> (value=w571:dbl)  [unwired: 1 in, 1 out]
                          n194 = Bundle By Name(cluster=w575, "Step Size [V]"=w571) -> (w574:T4)
                        }
                        frame 5 {
                          n195 = Decimal String To Number(string=w578) -> (number=w577:i32)  [unwired: 2 in, 1 out]
                          n196 = Bundle By Name(cluster=w580, "Step Interval [s]"=w577) -> (w579:T4)
                        }
                        frame 6 {
                          n197 = Decimal String To Number(string=w583) -> (number=w582:i32)  [unwired: 2 in, 1 out]
                          n198 = Bundle By Name(cluster=w585, "Number Of Steps"=w582) -> (w584:T4)
                        }
                        frame 7 {
                          n199 = Decimal String To Number(string=w588) -> (number=w587:i32)  [unwired: 2 in, 1 out]
                          n200 = Bundle By Name(cluster=w590, "AC frequency [Hz]"=w587) -> (w589:T4)
                        }
                        frame 8 {
                          w595 = u16 0 items=["serial", "parallel"] ("RC Configuration")
                          w594 = u16 1 items=["serial", "parallel"] ("RC Configuration")
                          n201 = Equal?(x=w596, y="serial") -> (x = y?=w593:bool)
                          n202 = Select(t=w595, s=w593, f=w594) -> (s? t:f=w592:u16)
                          n203 = Bundle By Name(cluster=w599, "RC Configuration"=w592) -> (w598:T4)
                        }
                        frame 9 {
                          n204 = Scan Value(string=w605, format string="%.1f") -> (value=w602:dbl)  [unwired: 1 in, 1 out]
                          n205 = Bundle By Name(cluster=w603, "AC amplitude [V]"=w602) -> (w601:T4)
                        }
                        frame 10 {
                          n206 = Scan Value(string=w608, format string="%.1f") -> (value=w607:dbl)  [unwired: 1 in, 1 out]
                          n207 = Bundle By Name(cluster=w611, "Ramp down steps [V]"=w607) -> (w610:T4)
                        }
                        frame 11 {
                          n208 = Decimal String To Number(string=w614) -> (number=w613:i32)  [unwired: 2 in, 1 out]
                          n209 = Bundle By Name(cluster=w616, "Ramp down Interval [s]"=w613) -> (w615:T4)
                        }
                        frame 12 {
                          n210 = case shown="False" w617 {
                            tunnel: w621 -> [w629 w630]
                            tunnel: [w628 w630] -> w620
                            tunnel: w619 -> [w627 _]
                            frame False {
                              n211 = Equal?(x=w627, y="Arduino") -> (x = y?=w625:bool)
                              n212 = Select(t=enum16{"Read Arduino", "Enter manually"}."Read Arduino" ("Temperature Readout"), s=w625, f=enum16{"Read Arduino", "Enter manually"}."Enter manually" ("Temperature Readout")) -> (s? t:f=w622:enum16{"Read Arduino", "Enter manually"})
                              n213 = Bundle By Name(cluster=w629, "Temperature Readout"=w622) -> (w628:T4)
                            }
                            frame True {
                            }
                          }
                        }
                        frame 13 {
                          n214 = Scan From String(format string="%f", input string=w635, error in=w631) -> (error out=w632:errorcluster, output 1=w637:dbl)  [unwired: 2 in, 2 out]
                          n215 = Bundle By Name(cluster=w634, "C_is Limit [pF/cm]"=w637) -> (w633:T4)
                        }
                      }
                    }
                  }
                }
              }
              n216 = call <vilib>:"Close File+.vi"("error in (no error)"=w478, "refnum"=w479) -> ()  [unwired: 3 in, 3 out]
            }
            frame Error {
              n217 = One Button Dialog(message="Can't open definitions file!") -> ()  [unwired: 1 in, 1 out]
            }
          }
          n218 = global write "QC_MeasurementSetup.vi" "Cis Measurement Parameters"(w467) -> ()
        }
        frame #4 {
          w650 = string[] ["BIASSUPPLY", "SMU", "LCR", "BIASV", "BASEV", "BASERAMP", "BASEINT", "HIGHV", "HIGHRAMP", "HIGHINT", "ACFREQUENCY", "RCCONFIG", "ACAMPLITUDE", "TREADOUT", "GOODSTRIPS", "CARD"]  # Keywords
          # "Read config from file"
          # "STRIPTEST"
          n219 = global read "QC_MeasurementSetup.vi" "Striptest Measurement Parameters"() -> (w642:T5)
          n220 = Current VI's Path() -> (path=w645:path)
          n221 = Strip Path(path=w645) -> (stripped path=w644:path)  [unwired: 1 out]
          n222 = Build Path(base path=w644, name or relative path=path "STRIPTESTconfig.txt") -> (appended path=w640:path)
          "Configuration File Striptest" <- w640
          n223 = Array Size(array=w650) -> (size(s)=w649:i32)
          n224 = call <vilib>:"Open File+.vi"("file path (\" \")"=w640) -> ("error out"=w646:errorcluster, "refnum"=w647:refnum<file>)  [unwired: 7 in, 2 out]
          n225 = case shown="No Error" w646 {
            selector: w646 -> [w652 _]
            tunnel: w647 -> [w659 _]
            tunnel: w650 -> [w658 _]
            tunnel: w649 -> [w657 _]
            tunnel: w642 -> [w656 w832]
            tunnel: [w655 w832] -> w643
            tunnel: w641 -> [w651 _]
            frame No Error {
              n226 = while {
                shift-left: w656 -> [w666]
                shift-right: [w664] -> w655
                tunnel: w657 -> [w663]
                tunnel: w658 -> [w669]
                tunnel: [w674] -> w654
                tunnel: w659 -> [w680]
                shift-right: [w661] -> w653
                shift-left: w652 -> [w673]
                tunnel: w651 -> [w660]
                stop <- w676 continue-if-true
                n227 = call <vilib>:"Read File+ (string).vi"("count"=0, "line mode (characters:F)"=TRUE, "error in (no error)"=w673, "refnum"=w680) -> ("error out"=w662:errorcluster, "string"=w675:string, "dup refnum"=w674:refnum<file>, "EOF?"=w678:bool)  [unwired: 3 in, 1 out]
                n228 = Unbundle By Name(w662) -> ("status"=w677:bool)
                n229 = Search/Split String(string=w675, search string/char (-)="%" ("search char (-)")) -> (substring before match=w668:string, match + rest of string=w681:string)  [unwired: 1 in, 1 out]
                n230 = Not Or(1:w678, 2:w677) -> (0:w676:bool)
                n231 = String Length(string=w681) -> (length=w667:i32)
                n232 = Subtract(x=w667, y=3) -> (x-y=w670:i32)
                n233 = String Subset(string=w681, offset (0)=1, length (rest)=w670) -> (substring=w665:string)
                n234 = for {
                  N: w663 -> [_]
                  tunnel: w669 -> [w693] mode=indexing
                  tunnel: w668 -> [w688]
                  shift-right: [w689] -> w664
                  shift-left: w666 -> [w690]
                  tunnel: w665 -> [w687]
                  shift-right: [w685] -> w661
                  shift-left: w662 -> [w686]
                  tunnel: w660 -> [w684]
                  i -> [w691]
                  n235 = Match Pattern(string=w693, regular expression=w688) -> (offset past match=w694:i32)  [unwired: 1 in, 3 out]
                  n236 = Increment(x=w694) -> (x+1=w695:i32)
                  n237 = Greater Than 0?(x=w695) -> (x > 0?=w692:bool)
                  n238 = case shown="True" w692 {
                    tunnel: w691 -> [_ w704]
                    tunnel: w687 -> [_ w703]
                    tunnel: w690 -> [w697 w702]
                    tunnel: [w697 w701] -> w689
                    tunnel: w686 -> [w696 w700]
                    tunnel: [w696 w699] -> w685
                    tunnel: w684 -> [_ w698]
                    frame False {
                    }
                    frame True {
                      n239 = case shown="14" w704 {
                        tunnel: w703 -> [w708 w724 w738 w750 w756 w762 w766 w773 w779 w783 w788 w797 w802 w809 w824 w828]
                        tunnel: w702 -> [w707 w723 w737 w752 w758 w764 w769 w770 w776 w784 w789 w800 w805 w811 w823 w831]
                        tunnel: [w715 w729 w743 w751 w757 w763 w768 w771 w777 w785 w790 w799 w804 w810 w821 w829] -> w701
                        tunnel: w700 -> [w713 w728 w742 w747 w753 w759 w767 w772 w778 w786 w791 w792 w801 w808 w822 w830]
                        tunnel: [w714 w727 w741 w747 w753 w759 w767 w772 w778 w786 w791 w792 w801 w808 w822 w830] -> w699
                        tunnel: w698 -> [w706 w721 w735 _ _ _ _ _ _ _ _ _ _ w807 _ _]
                        frame 0, Default {
                          n240 = case shown="True" w706 {
                            tunnel: w708 -> [w716 _]
                            tunnel: [w716 w717] -> w705
                            tunnel: w707 -> [_ w718]
                            frame False {
                            }
                            frame True {
                              n241 = Unbundle By Name(w718) -> ("Bias Supply Name"=w717:string)
                            }
                          }
                          n242 = call "InstrumentSelection.vi"("error in (no error)"=w713, "Verify GPIB address"=FALSE, "Instrument type"=enum16{"Supply", "LCR", "Multimeter"}."Supply", "Instrument name IN"=w705) -> ("error out"=w714:errorcluster, "Instrument name OUT"=w709:string, "Supply"=w712:refnum<class "SupplyControl.lvclass">)  [unwired: 2 in, 3 out]
                          n243 = Bundle By Name(cluster=w707, "Bias Supply"=w712, "Bias Supply Name"=w709) -> (w715:T5)
                        }
                        frame 1 {
                          n244 = case shown="True" w721 {
                            tunnel: w724 -> [w730 _]
                            tunnel: [w730 w731] -> w722
                            tunnel: w723 -> [_ w732]
                            frame False {
                            }
                            frame True {
                              n245 = Unbundle By Name(w732) -> ("SMU Name"=w731:string)
                            }
                          }
                          n246 = call "InstrumentSelection.vi"("error in (no error)"=w728, "Verify GPIB address"=FALSE, "Instrument type"=enum16{"Supply", "LCR", "Multimeter"}."Supply", "Instrument name IN"=w722) -> ("error out"=w727:errorcluster, "Instrument name OUT"=w726:string, "Supply"=w719:refnum<class "SupplyControl.lvclass">)  [unwired: 2 in, 3 out]
                          n247 = Bundle By Name(cluster=w723, "SMU"=w719, "SMU Name"=w726) -> (w729:T5)
                        }
                        frame 2 {
                          n248 = case shown="True" w735 {
                            tunnel: w738 -> [w744 _]
                            tunnel: [w744 w745] -> w736
                            tunnel: w737 -> [_ w746]
                            frame False {
                            }
                            frame True {
                              n249 = Unbundle By Name(w746) -> ("LCR Name"=w745:string)
                            }
                          }
                          n250 = call "InstrumentSelection.vi"("error in (no error)"=w742, "Verify GPIB address"=FALSE, "Instrument type"=enum16{"Supply", "LCR", "Multimeter"}."LCR", "Instrument name IN"=w736) -> ("error out"=w741:errorcluster, "Instrument name OUT"=w740:string, "LCR"=w733:refnum<class "LCRControl.lvclass">)  [unwired: 2 in, 3 out]
                          n251 = Bundle By Name(cluster=w737, "LCR"=w733, "LCR Name"=w740) -> (w743:T5)
                        }
                        frame 3 {
                          n252 = Scan Value(string=w750, format string="%.1f") -> (value=w749:dbl)  [unwired: 1 in, 1 out]
                          n253 = Bundle By Name(cluster=w752, "Bias Voltage [V]"=w749) -> (w751:T5)
                        }
                        frame 4 {
                          n254 = Scan Value(string=w756, format string="%.1f") -> (value=w755:dbl)  [unwired: 1 in, 1 out]
                          n255 = Bundle By Name(cluster=w758, "Base Voltage [V]"=w755) -> (w757:T5)
                        }
                        frame 5 {
                          n256 = Scan Value(string=w762, format string="%.1f") -> (value=w761:dbl)  [unwired: 1 in, 1 out]
                          n257 = Bundle By Name(cluster=w764, "Base Ramp Step [V]"=w761) -> (w763:T5)
                        }
                        frame 6 {
                          n258 = Decimal String To Number(string=w766) -> (number=w765:i32)  [unwired: 2 in, 1 out]
                          n259 = Bundle By Name(cluster=w769, "Base Ramp Interval [ms]"=w765) -> (w768:T5)
                        }
                        frame 7 {
                          n260 = Scan Value(string=w773, format string="%.1f") -> (value=w775:dbl)  [unwired: 1 in, 1 out]
                          n261 = Bundle By Name(cluster=w770, "High Voltage [V]"=w775) -> (w771:T5)
                        }
                        frame 8 {
                          n262 = Scan Value(string=w779, format string="%.1f") -> (value=w781:dbl)  [unwired: 1 in, 1 out]
                          n263 = Bundle By Name(cluster=w776, "High Ramp Step [V]"=w781) -> (w777:T5)
                        }
                        frame 9 {
                          n264 = Decimal String To Number(string=w783) -> (number=w782:i32)  [unwired: 2 in, 1 out]
                          n265 = Bundle By Name(cluster=w784, "High Ramp Interval [ms]"=w782) -> (w785:T5)
                        }
                        frame 10 {
                          n266 = Decimal String To Number(string=w788) -> (number=w787:i32)  [unwired: 2 in, 1 out]
                          n267 = Bundle By Name(cluster=w789, "AC frequency [Hz]"=w787) -> (w790:T5)
                        }
                        frame 11 {
                          w796 = u16 0 items=["serial", "parallel"] ("RC Configuration")
                          w795 = u16 1 items=["serial", "parallel"] ("RC Configuration")
                          n268 = Equal?(x=w797, y="serial") -> (x = y?=w794:bool)
                          n269 = Select(t=w796, s=w794, f=w795) -> (s? t:f=w793:u16)
                          n270 = Bundle By Name(cluster=w800, "RC Configuration"=w793) -> (w799:T5)
                        }
                        frame 12 {
                          n271 = Scan Value(string=w802, format string="%.1f") -> (value=w803:dbl)  [unwired: 1 in, 1 out]
                          n272 = Bundle By Name(cluster=w805, "AC amplitude [V]"=w803) -> (w804:T5)
                        }
                        frame 13 {
                          n273 = case shown="False" w807 {
                            tunnel: w811 -> [w819 w820]
                            tunnel: [w818 w820] -> w810
                            tunnel: w809 -> [w817 _]
                            frame False {
                              n274 = Equal?(x=w817, y="Arduino") -> (x = y?=w815:bool)
                              n275 = Select(t=enum16{"Read Arduino", "Enter manually"}."Read Arduino" ("Temperature Readout"), s=w815, f=enum16{"Read Arduino", "Enter manually"}."Enter manually" ("Temperature Readout")) -> (s? t:f=w812:enum16{"Read Arduino", "Enter manually"})
                              n276 = Bundle By Name(cluster=w819, "Temperature Readout"=w812) -> (w818:T5)
                            }
                            frame True {
                            }
                          }
                        }
                        frame 14 {
                          n277 = Scan Value(string=w824, format string="%.1f") -> (value=w825:dbl)  [unwired: 1 in, 1 out]
                          n278 = Bundle By Name(cluster=w823, "Fraction of good strips [%]"=w825) -> (w821:T5)
                        }
                        frame 15 {
                          n279 = Decimal String To Number(string=w828) -> (number=w827:i32)  [unwired: 2 in, 1 out]
                          n280 = Bundle By Name(cluster=w831, "Probe Card Channels"=w827) -> (w829:T5)
                        }
                      }
                    }
                  }
                }
              }
              n281 = call <vilib>:"Close File+.vi"("error in (no error)"=w653, "refnum"=w654) -> ()  [unwired: 3 in, 3 out]
            }
            frame Error {
              n282 = One Button Dialog(message="Can't open definitions file!") -> ()  [unwired: 1 in, 1 out]
            }
          }
          n283 = global write "QC_MeasurementSetup.vi" "Striptest Measurement Parameters"(w643) -> ()
        }
      }
    }
  }
